vi "validate control references.vi"(8 "error in (no error)":errorcluster, 9 "VI Name":string, 10 "front panel elements in":refnum<vi>[](array[refnum]), 11 "channels in":refnum<class "TBM channel.lvclass">[](array[class])) -> (0 "error out":errorcluster)   [LabVIEW 2015, in "UI Reference runtime.lvclass"]
uses:
  UI Reference runtime.lvclass
  <vilib>/NI/Tag Bus Module Framework/channel/TBM channel.lvclass
  <vilib>/NI/Tag Bus Module Framework/channel/TBM channel.lvclass/TBM channel.ctl
  <vilib>/NI/Tag Bus/tag/tag descriptor.lvclass/tag descriptor.ctl
  <vilib>/NI/Tag Bus Module Framework/channel/Read channel classification.vi
  <vilib>/NI/Tag Bus/tag/read tag name.vi
  <vilib>/NI/Tag Bus/tag/read data type.vi
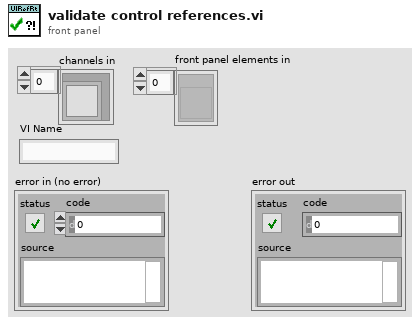
[diagram p1: front panel]
types:
  T1 = typedef "TBM channel.lvclass/channel classification.ctl" = enum16{"input data", "output data", "processing parameter", "processing result"}
  T2 = typedef "tag bus.lvlib/tag descriptor.lvclass/Data Type.ctl" = enum16{"Double", "Single", "I64", "I32", "I16", "I8", "U64", "U32", "U16", "U8", "Boolean", "String", "Array of Double", "Array of Single", "Array of I64", "Array of I32", "Array of I16", "Array of I8", "Array of U64", "Array of U32", "Array of U16", "Array of U8", "Array of Boolean", "Array of String"}
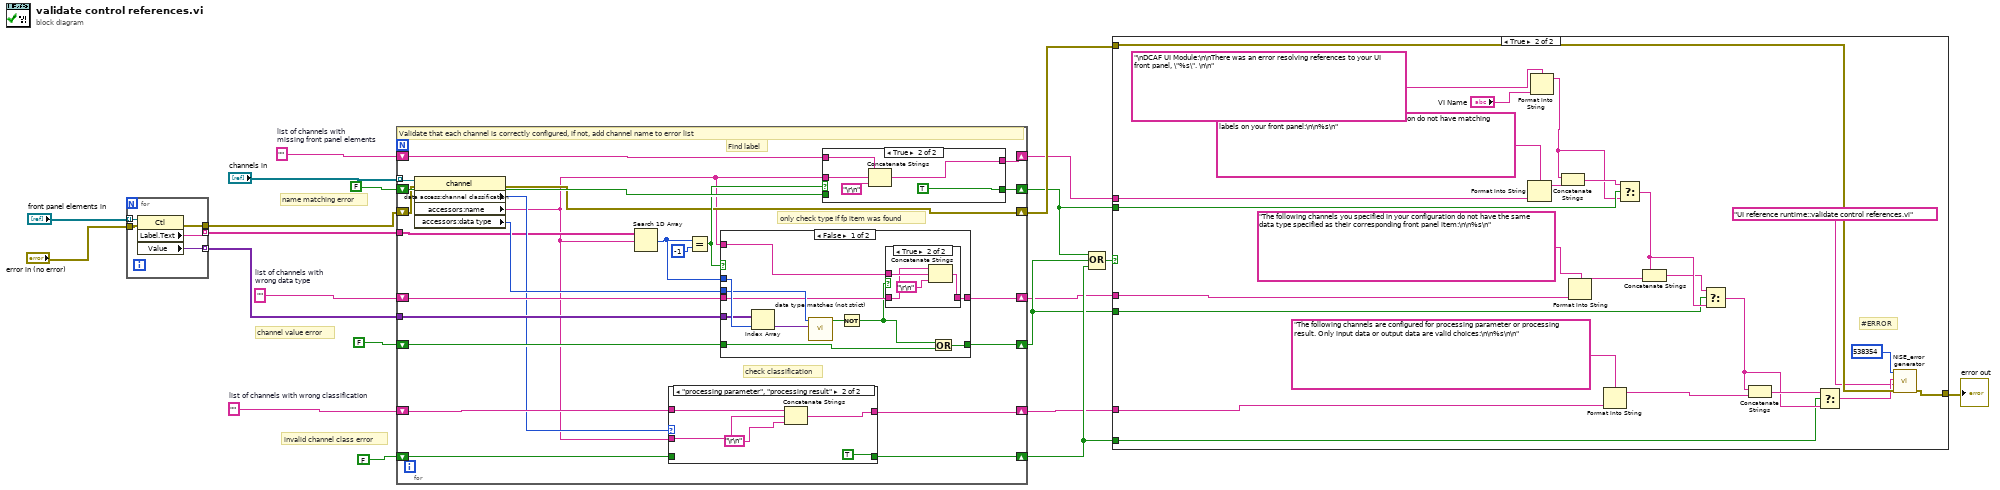
[diagram p0: block diagram]
diagram:
  w12 = ""  # list of channels with  wrong data type
  w10 = ""  # list of channels with wrong classification
  w7 = ""  # list of channels with  missing front panel elements
  # "channel value error"
  # "invalid channel class error"
  # "name matching error"
  n1 = for {
    tunnel: "front panel elements in" -> [w26] mode=indexing
    tunnel: [w25] -> w4 mode=indexing
    tunnel: [w24] -> w3 mode=indexing
    tunnel: "error in (no error)" -> [w23]
    tunnel: [w22] -> w1
    n2 = property class="Ctl"(reference=w26, error in=w23) -> (error out=w22:errorcluster, "Label.Text"=w25:string, "Value"=w24:variant)  [unwired: 1 out]
  }
  n3 = for {
    tunnel: "channels in" -> [w49] mode=indexing
    shift-right: [w47] -> w14
    shift-left: w7 -> [w48]
    shift-right: [w46] -> w17
    shift-left: FALSE -> [w45]
    shift-right: [w43] -> w19
    shift-left: FALSE -> [w44]
    shift-right: [w41] -> w16
    shift-left: w10 -> [w42]
    tunnel: w4 -> [w28]
    tunnel: w3 -> [w34]
    shift-right: [w37] -> w18
    shift-left: FALSE -> [w38]
    shift-right: [w32] -> w15
    shift-left: w12 -> [w33]
    shift-right: [w29] -> w21
    shift-left: w1 -> [w30]
    # "check classification"
    # "only check type if fp item was found"
    # "Find label"
    # "Validate that each channel is correctly configured, if not, add channel name to error list"
    n4 = property class="channel"(reference=w49, error in=w30) -> (error out=w29:errorcluster, "data access:channel classification"=w31:T1, "accessors:name"=w27:string, "accessors:data type"=w35:T2)  [unwired: 1 out]
    n5 = Search 1D Array(1D array=w28, element=w27) -> (index of element=w36:i32)  [unwired: 1 in]
    n6 = case shown="\"processing parameter\", \"processing result\"" w31 {
      tunnel: w44 -> [w69 _]
      tunnel: [w69 TRUE] -> w43
      tunnel: w42 -> [w68 w73]
      tunnel: w27 -> [_ w72]
      tunnel: [w68 w71] -> w41
      frame Default {
      }
      frame "processing parameter", "processing result" {
        n7 = Concatenate Strings(w73, w72, "\r\n") -> (w71:string)
      }
    }
    n8 = Equal?(x=w36, y=-1) -> (x = y?=w39:bool)
    n9 = case shown="False" w39 {
      tunnel: w38 -> [w51 w67]
      tunnel: [w53 w67] -> w37
      tunnel: w36 -> [w60 _]
      tunnel: w35 -> [w58 _]
      tunnel: w34 -> [w50 _]
      tunnel: w33 -> [w56 w66]
      tunnel: w27 -> [w57 _]
      tunnel: [w55 w66] -> w32
      frame False {
        n10 = Index Array(array=w50, index=w60) -> (element=w59:variant)
        n11 = call "data type matches (not strict).vi"("Value"=w59, "data type"=w58) -> ("type match"=w54:bool)  [unwired: 8 in, 1 out]
        n12 = Not(x=w54) -> (.not. x?=w52:bool)
        n13 = case shown="True" w52 {
          tunnel: w57 -> [_ w65]
          tunnel: w56 -> [w61 w63]
          tunnel: [w61 w64] -> w55
          frame False {
          }
          frame True {
            n14 = Concatenate Strings(w63, w65, "\r\n") -> (w64:string)
          }
        }
        n15 = Or(x=w52, y=w51) -> (x .or. y?=w53:bool)
      }
      frame True {
      }
    }
    n16 = case shown="True" w39 {
      tunnel: w48 -> [w76 w81]
      tunnel: w27 -> [_ w80]
      tunnel: [w76 w79] -> w47
      tunnel: [w75 TRUE] -> w46
      tunnel: w45 -> [w75 _]
      frame False {
      }
      frame True {
        n17 = Concatenate Strings(w81, w80, "\r\n") -> (w79:string)
      }
    }
  }
  n18 = Compound Arithmetic op=OR(w17, w18, w19) -> (w13:bool)
  n19 = case shown="True" w13 {
    tunnel: w14 -> [_ w106]
    tunnel: w15 -> [_ w105]
    tunnel: w16 -> [_ w104]
    tunnel: w17 -> [_ w99]
    tunnel: w18 -> [_ w96]
    tunnel: w19 -> [_ w93]
    tunnel: [w82 w92] -> w20
    tunnel: w21 -> [w82 w91]
    frame False {
    }
    frame True {
      # "#ERROR"
      n20 = Format Into String(format string="The following channels you specified in your configuration do not have matching labels on your front panel:\n\n%s\n", w106) -> (resulting string=w103:string)  [unwired: 2 in, 1 out]
      n21 = Format Into String(format string="\nDCAF UI Module:\n\nThere was an error resolving references to your UI front panel, \"%s\". \n\n", "VI Name") -> (resulting string=w89:string)  [unwired: 2 in, 1 out]
      n22 = Concatenate Strings(w89, w103) -> (w100:string)
      n23 = Format Into String(format string="The following channels you specified in your configuration do not have the same data type specified as their corresponding front panel item:\n\n%s\n", w105) -> (resulting string=w102:string)  [unwired: 2 in, 1 out]
      n24 = Format Into String(format string="The following channels are configured for processing parameter or processing result. Only input data or output data are valid choices:\n\n%s\n\n", w104) -> (resulting string=w101:string)  [unwired: 2 in, 1 out]
      n25 = Select(t=w100, s=w99, f=w89) -> (s? t:f=w98:string)
      n26 = Concatenate Strings(w98, w102) -> (w97:string)
      n27 = Select(t=w97, s=w96, f=w98) -> (s? t:f=w94:string)
      n28 = Concatenate Strings(w94, w101) -> (w95:string)
      n29 = Select(t=w95, s=w93, f=w94) -> (s? t:f=w84:string)
      n30 = call <vilib>:"NISE_error generator.vi"("error in"=w91, "source"="UI reference runtime::validate control references.vi", "append error message"=w84, "error code (0)"=538354) -> ("error out"=w92:errorcluster)  [unwired: 5 in]
    }
  }
  "error out" <- w20
